vi "Big5toHex.vi"(1 "String":string) -> (0 "hex integer string":string[](array[string]))   [LabVIEW 2015]
panel:
  out "Array":string[](array[string])
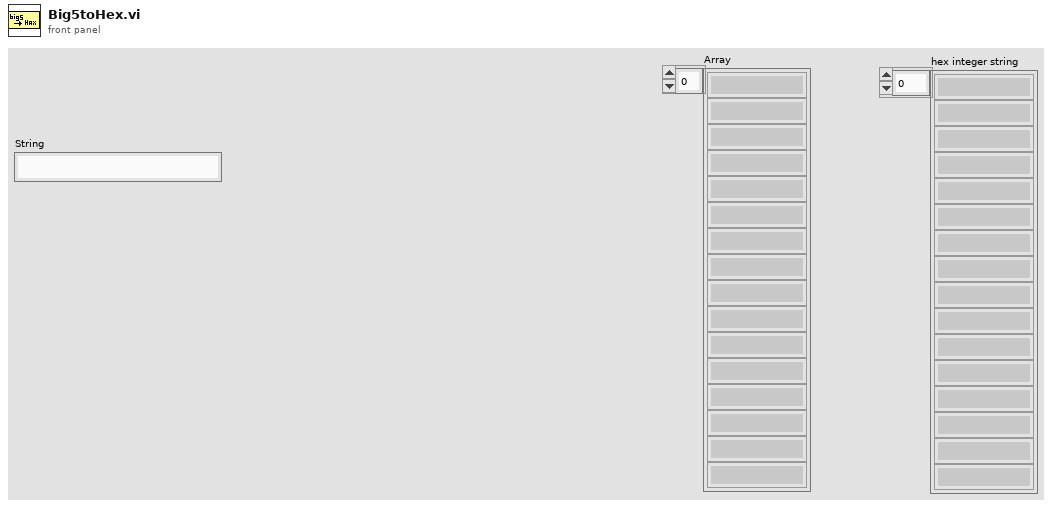
[diagram p1: front panel]
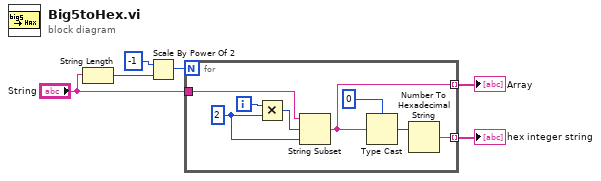
[diagram p0: block diagram]
diagram:
  n1 = String Length(string="String") -> (length=w6:i32)
  n2 = Scale By Power Of 2(n=-1, x=w6) -> (x*2^n=w4:i32)
  n3 = for {
    N: w4 -> [_]
    tunnel: "String" -> [w14]
    tunnel: [w8] -> w2 mode=indexing
    tunnel: [w7] -> w1 mode=indexing
    i -> [w13]
    w12 = 2 ("length (rest)")
    n4 = Multiply(x=w13, y=w12) -> (x*y=w11:i32)
    n5 = String Subset(string=w14, offset (0)=w11, length (rest)=w12) -> (substring=w7:string)
    n6 = Type Cast(type=u16 0, x=w7) -> (*(type *) &x=w10:u16)
    n7 = Number To Hexadecimal String(2:w10) -> (0:w8:string)  [unwired: 1 in]
  }
  "Array" <- w1
  "hex integer string" <- w2
